vi "Data Producer Worker Template_Stop.vi"(0 "Data Producer Worker Template In":refnum<class "Data Producer Worker Template.lvclass">, 11 "error in (no error)":errorcluster) -> (15 "error out":errorcluster)   [LabVIEW 2013, in "Data Producer Worker Template.lvclass"]
uses:
  Data Producer Worker Template.lvclass
  Data Producer Worker Template.lvclass/Data Producer Worker Template.ctl
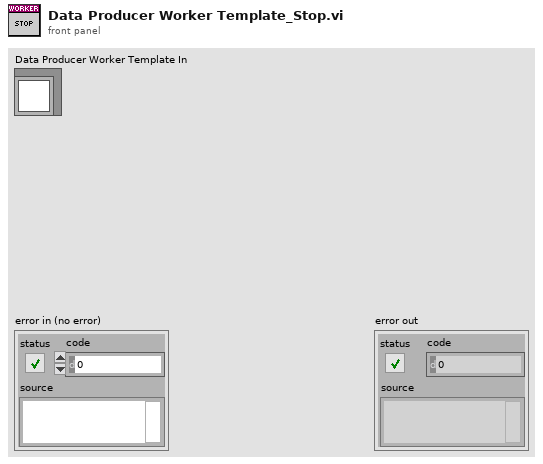
[diagram p1: front panel]
types:
  T1 = typedef "Data Producer Worker Template.lvclass/Data Producer Worker Template_Data Queue.ctl" = refnum<queue>
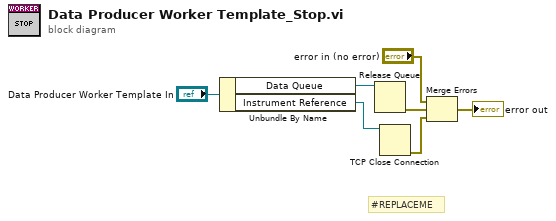
[diagram p0: block diagram]
diagram:
  # "#REPLACEME"
  n1 = Unbundle By Name("Data Producer Worker Template In") -> ("Data Queue"=w6:T1, "Instrument Reference"=w2:refnum<k5>)
  n2 = Release Queue(queue=w6) -> (error out=w5:errorcluster)  [unwired: 2 in, 2 out]
  n3 = TCP Close Connection(connection ID=w2) -> (error out=w1:errorcluster)  [unwired: 2 in, 1 out]
  n4 = Merge Errors("error in (no error)", w5, w1) -> (→"error out":errorcluster)
